vi "Impedence Transform.vi"(11 "input impedance":u32(ring) items=["1 mega ohm"=0, "50 ohms"=2]) -> (3 "Impedance":dbl)   [LabVIEW 2019, in "5105.lvlib" / "5105.lvclass"]
uses:
  5105.lvclass
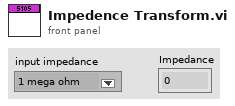
[diagram p1: front panel]
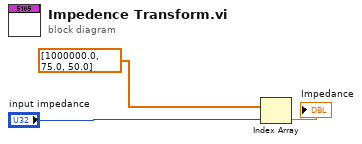
[diagram p0: block diagram]
diagram:
  n1 = Index Array(array=dbl[] [1000000.0, 75.0, 50.0] ("input impedance arr"), index="input impedance") -> (element=→"Impedance":dbl)
